vi "determineSubDataSVs.vi"(8 "error in (no error)":errorcluster, 11 "MiddlewareSVThisComponent in":refnum<class "MiddlewareSVThisComponent.lvclass">) -> (0 "error out":errorcluster, 2 "svNames":string[](array[string]), 3 "MiddlewareSVThisComponent out":refnum<class "MiddlewareSVThisComponent.lvclass">)   [LabVIEW 2015, in "MiddlewareSVThisComponent.lvclass"]
uses:
  MiddlewareSVThisComponent.lvclass
  Typedefs/SubDataSV.ctl
  MiddlewareSVThisComponent.lvclass/MiddlewareSVThisComponent.ctl
  Typedefs/EXATypedefs.lvlib
  <vilib>/Utility/Data Type/NI_Data Type.lvlib
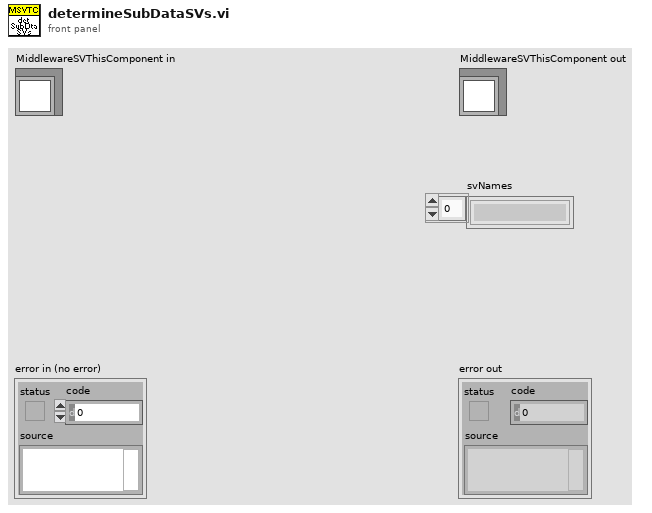
[diagram p1: front panel]
types:
  T1 = typedef "EXATypedefs.lvlib/SubDataSV.ctl" = enum16{"ClearError", "Disable", "Enable", "Exit", "GoToStandby", "HeartbeatIn", "Start"}
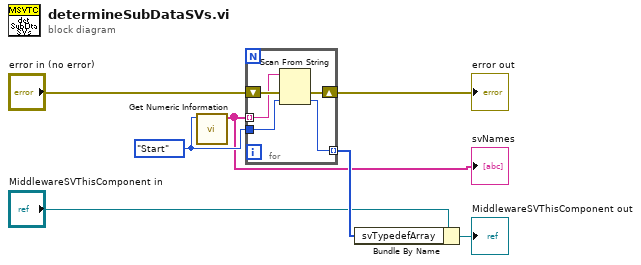
[diagram p0: block diagram]
diagram:
  w4 = SubDataSV."Start" ("SubDataSV")
  n1 = call <vilib>:"Get Numeric Information.vi"("Variant"=w4) -> ("Enum Names"=w3:string[])  [unwired: 7 in, 3 out]
  "svNames" <- w3
  n2 = for {
    tunnel: [w11] -> w7 mode=indexing
    shift-right: [w9] -> w1
    shift-left: "error in (no error)" -> [w10]
    tunnel: w3 -> [w8] mode=indexing
    tunnel: w4 -> [w12]
    n3 = Scan From String(input string=w8, error in=w10, default 1=w12) -> (error out=w9:errorcluster, output 1=w11:T1)  [unwired: 2 in, 2 out]
  }
  "error out" <- w1
  n4 = Bundle By Name(cluster="MiddlewareSVThisComponent in", "svTypedefArray"=w7) -> (→"MiddlewareSVThisComponent out":refnum<class "MiddlewareSVThisComponent.lvclass">)
